vi "Measure Multiple.vi"(8 "error in (no error)":errorcluster, 11 "NI SMU in":refnum<class "NI SMU.lvclass">) -> (0 "error out":errorcluster, 2 "Data":variant, 3 "NI SMU out":refnum<class "NI SMU.lvclass">)   [LabVIEW 2020, in "NI SMU.lvlib" / "NI SMU.lvclass"]
uses:
  NI SMU.lvclass
  NI SMU.lvclass/NI SMU.ctl
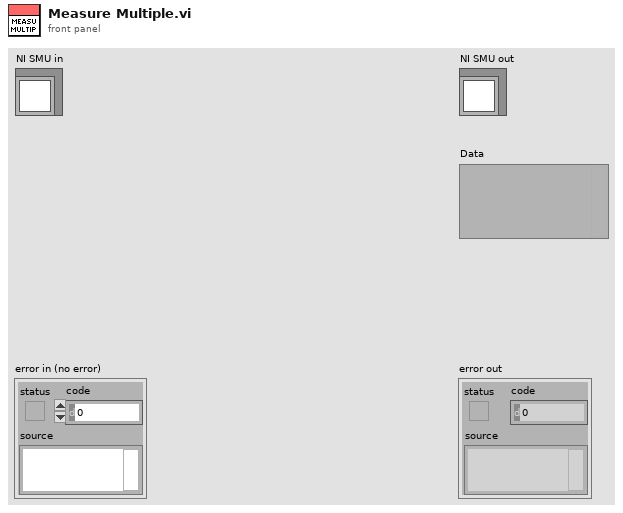
[diagram p1: front panel]
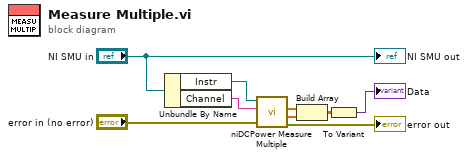
[diagram p0: block diagram]
diagram:
  n1 = Unbundle By Name("NI SMU in") -> ("Instr"=w8:refnum<k15>, "Channel"=w9:string)
  n2 = call <instrlib>:"niDCPower Measure Multiple.vi"("error in (no error)"="error in (no error)", "channel name"=w9, "instrument handle"=w8) -> ("error out"=→"error out":errorcluster, "current measurements"=w3:dbl[], "voltage measurements"=w4:dbl[])  [unwired: 5 in, 1 out]
  n3 = Build Array(w4, w3) -> (w2:dbl[][])
  n4 = To Variant(anything=w2) -> (Variant=→"Data":variant)
  "NI SMU out" <- "NI SMU in"
